vi "总磷氨氮测量流程.vi"(10 "量程模式":T1, 11 "参数":T2={"站号"=1, "量程切换"=enum."AUTO", "控制命令"=enum."启动测量", "模式设置"=enum."待机", "测量间隔"=0} {"站号" items=["总磷"=1, "总氮"=2]}) -> ()   [LabVIEW 2016]
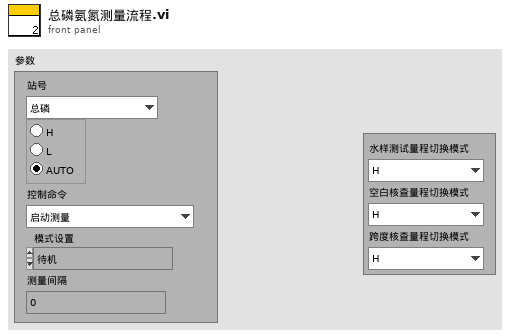
[diagram p1: front panel]
types:
  T1 = cluster{"水样测试量程切换模式":enum16{"H", "L", "AUTO"}, "空白核查量程切换模式":enum16{"H", "L", "AUTO"}, "跨度核查量程切换模式":enum16{"H", "L", "AUTO"}}
  T2 = cluster{"站号":u16, "量程切换":enum32{"H", "L", "AUTO"}, "控制命令":enum16{"启动测量", "标样核查", "零点核查", "跨度核查", "空白测试", "平行样测试", "加标回收", "空白校准", "标样校准", "初始化（清洗）", "停止测试", "仪器重启", "校时", "模式设置", "测量间隔设置"}, "模式设置":enum16{"待机", "连续模式", "周期模式", "定点模式", "受控模式", "手动模式"}, "测量间隔":u16}
  T3 = enum16{"初始化", "通电", "参数1启动", "等待参数1测试完成", "参数1测试完成", "参数1存储数据", "参数2启动", "等待参数2测试完成", "参数2测试完成", "参数2存储数据", "断电", "结束"}
  T4 = cluster{"时间标识":timestamp, "设备":string, "日志信息":string, "流程参数":string}
  T5 = cluster{"时间标识":timestamp, "监测值":sgl, "单位":u16, "数据标识":string, "因子编码":u32, "标样参考值":sgl, "F0":sgl, "F1":sgl, "F2":sgl, "F3":sgl, "温度":sgl, "湿度":sgl, "量程标识":string}
  T6 = enum16{"维护数据", "水样测试", "标样核查", "零点核查", "跨度核查", "空白测试", "平行样测试", "加标回收", "空白校准", "标样校准", "初始化（清洗）"}
  T7 = cluster{"系统时间":timestamp, "工作状态":enum16{"空闲", "水样测试", "标样核查", "零点核查", "跨度核查", "空白测试", "平行样测试", "加标回收", "空白校准", "标样校准", "初始化（清洗）"}, "测量模式":enum16{"待机", "连续模式", "周期模式", "定点模式", "受控模式", "手动模式"}, "告警代码":enum16{"无告警", "缺试剂告警", "缺水样告警", "缺蒸馏水告警", "缺标液告警", "仪表漏液告警", "标定异常告警", "超量程告警", "加热异常", "低试剂预警", "超上限告警", "超下限告警", "仪表内部其他异常", "滴定异常告警", "电极异常告警", "量程切换告警", "参数设置告警", "PH电极电位异常", "电导率电极异常", "浊度光度异常", "溶解氧电极异常", "溶解氧光强异常", "温度异常告警", "PH异常告警", "溶解氧异常告警", "电导率异常告警", "浊度异常告警", "叶绿素异常告警", "藻密度异常告警", "蓝绿藻异常告警", "ORP异常告警", "氨氮异常告警", "清洁刷异常告警", "SD卡异常告警", "蓝牙异常告警", "Wifi异常告警", "流程异常告警"}, "故障代码":enum16{"无故障", "电机故障", "温度故障", "通讯故障", "滴定故障"}, "日志代码":u16, "软件版本":u16, "F0":sgl, "F1":sgl, "F2":sgl, "F3":sgl, "T":sgl, "H":sgl, "id":u16, "flowid":u16, "量程":u16, "总磷控温温度1":sgl, "营养盐控温温度2":sgl, "ADC":sgl}
  T8 = enum16{"启动测量", "标样核查", "零点核查", "跨度核查", "空白测试", "平行样测试", "加标回收", "空白校准", "标样校准", "初始化（清洗）", "停止测试", "仪器重启", "校时", "模式设置", "测量间隔设置"}
  T9 = enum16{"空闲", "水样测试", "标样核查", "零点核查", "跨度核查", "空白测试", "平行样测试", "加标回收", "空白校准", "标样校准", "初始化（清洗）"}
  T10 = cluster{"因子编码":u32, "单位":u16, "标样参考值":sgl, "水样数据时间":timestamp, "水样实测值":sgl, "水样数据标识":string, "标样数据时间":timestamp, "标样实测值":sgl, "标样数据标识":string, "空白数据时间":timestamp, "空白实测值":sgl, "空白数据标识":string, "零点核查数据时间":timestamp, "零点核查实测值":sgl, "零点核查数据标识":string, "跨度核查数据时间":timestamp, "跨度核查实测值":sgl, "跨度核查数据标识":string, "加标回收数据时间":timestamp, "加标回收实测值":sgl, "加标回收数据标识":string, "平行样数据时间":timestamp, "平行样实测值":sgl, "平行样数据标识":string}
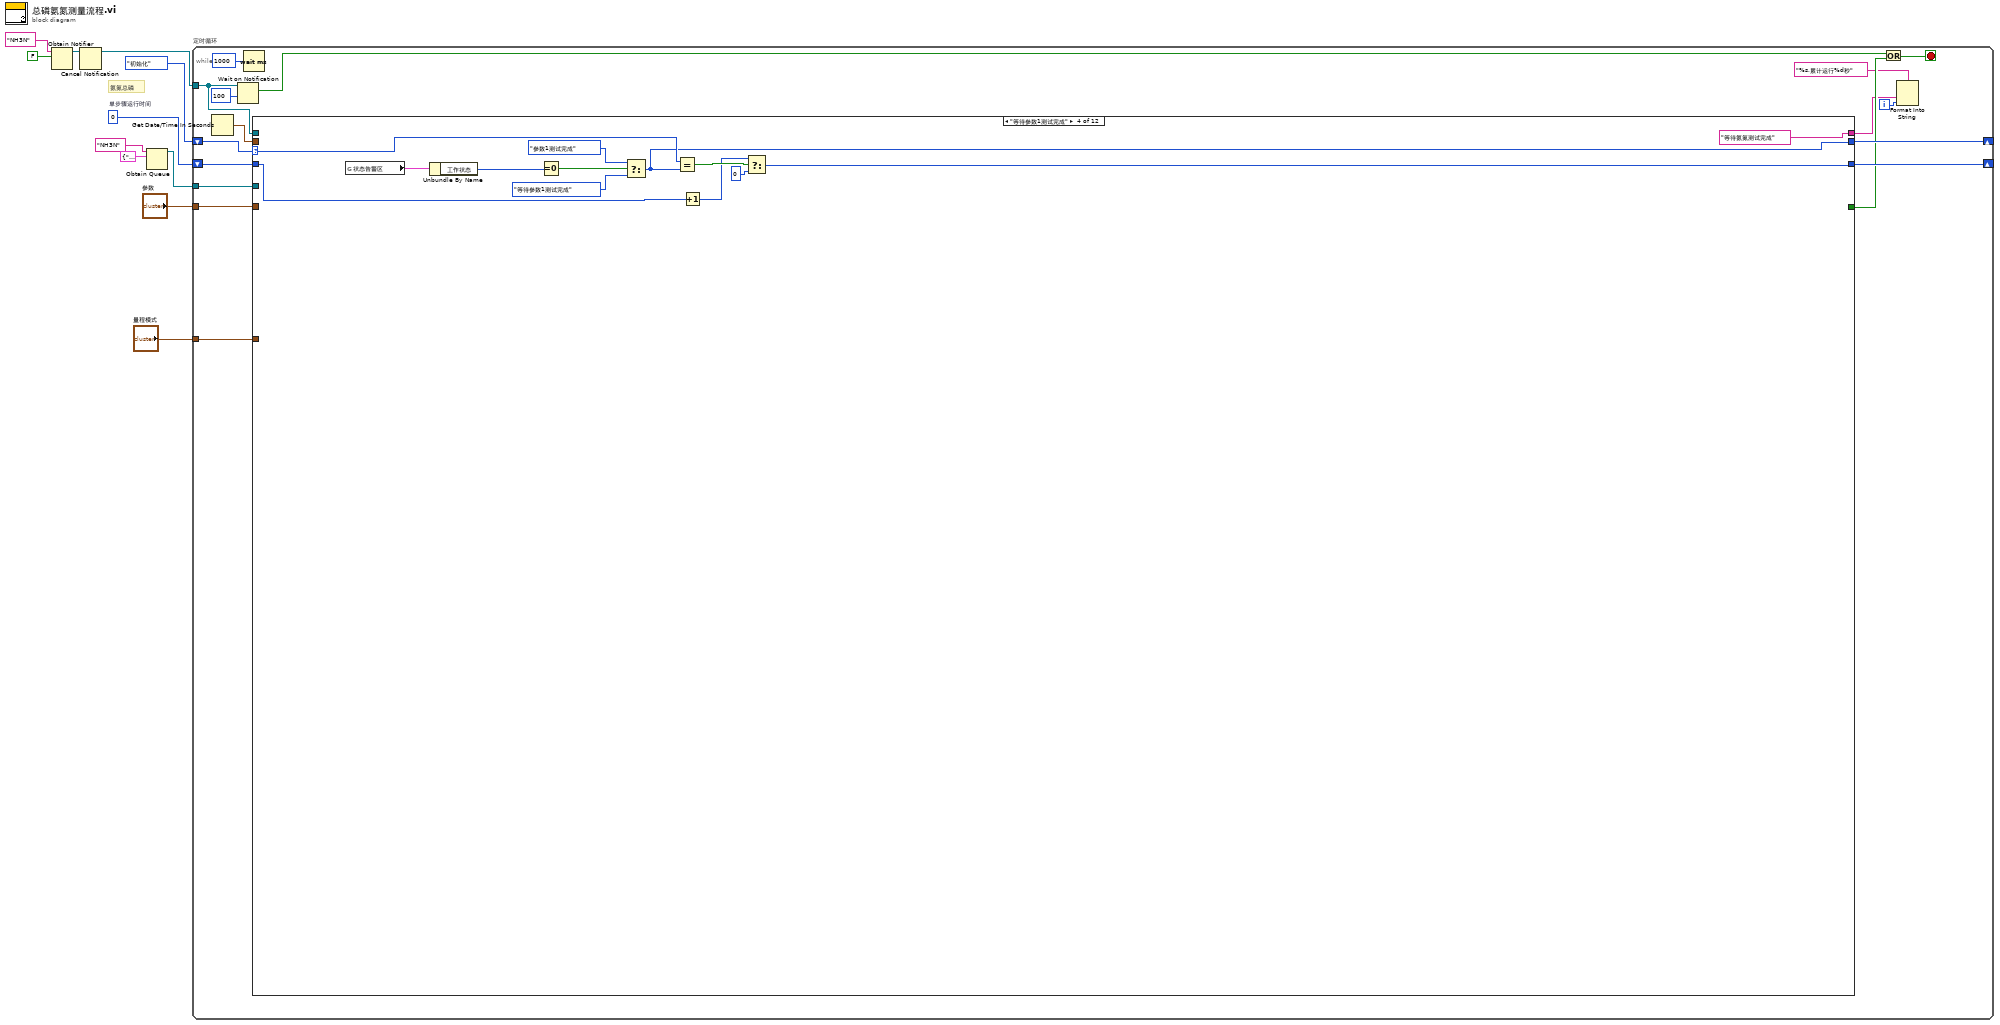
[diagram p0: block diagram]
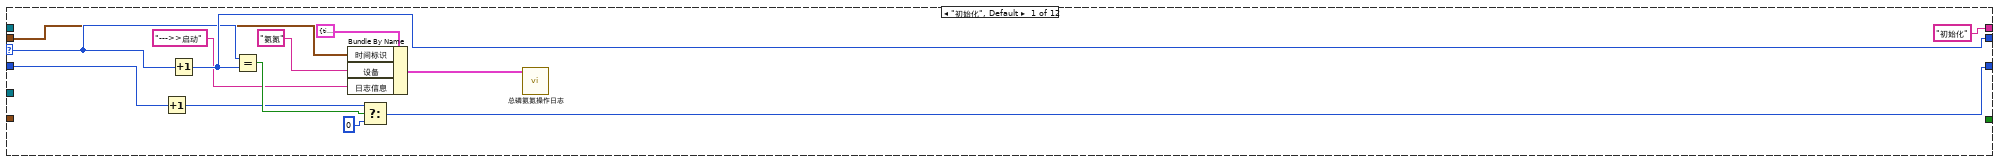
[diagram p2: hidden frame]
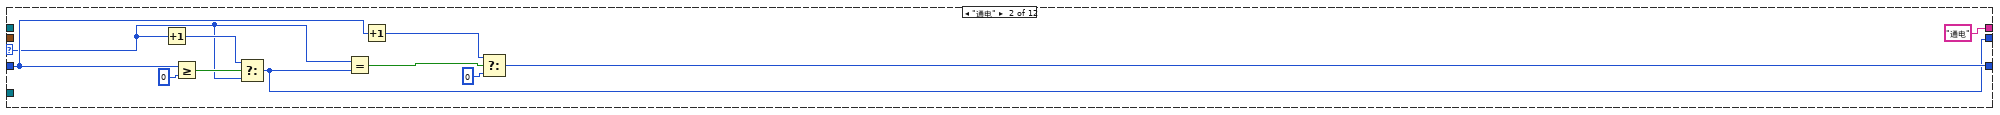
[diagram p3: hidden frame]
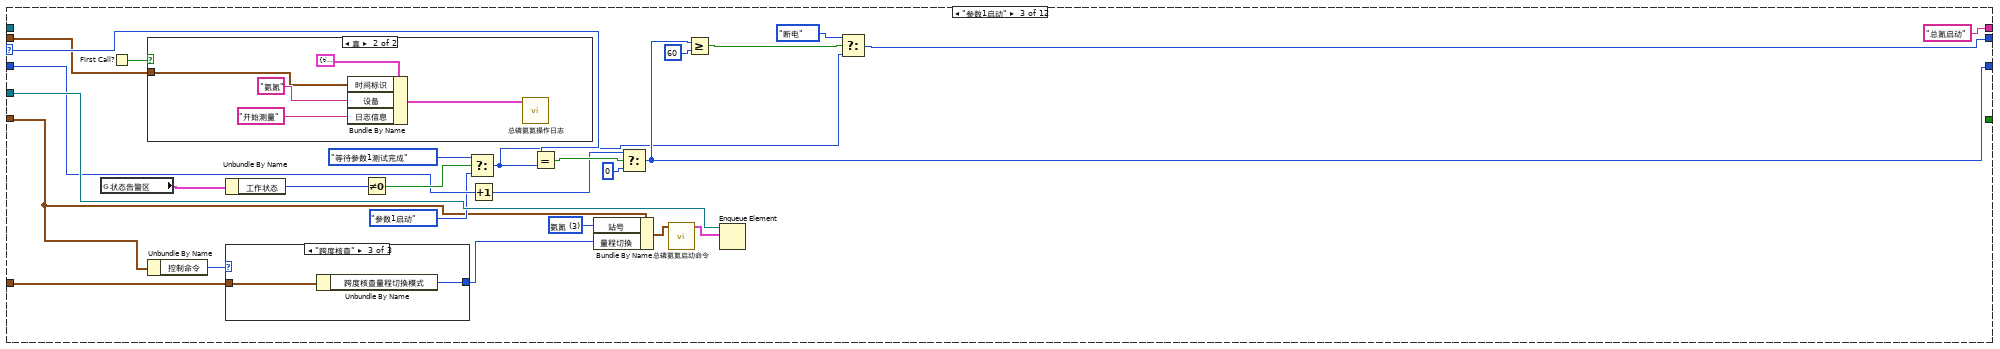
[diagram p4: hidden frame]
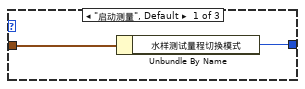
[diagram p5: hidden frame]
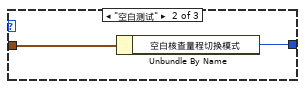
[diagram p6: hidden frame]
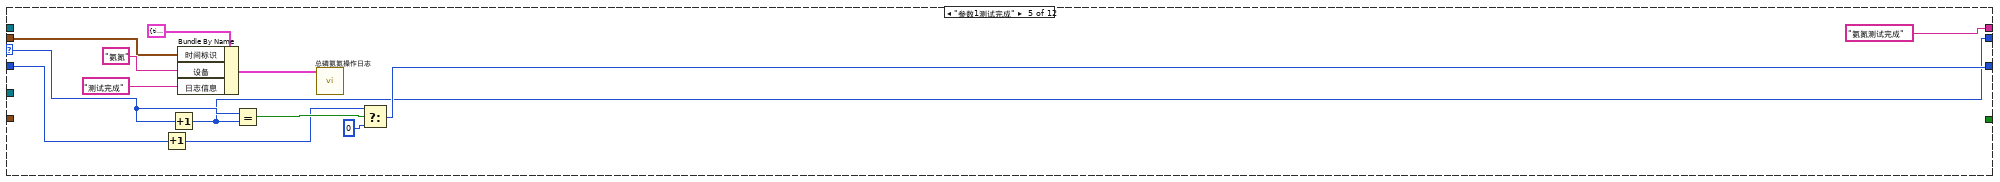
[diagram p8: hidden frame]
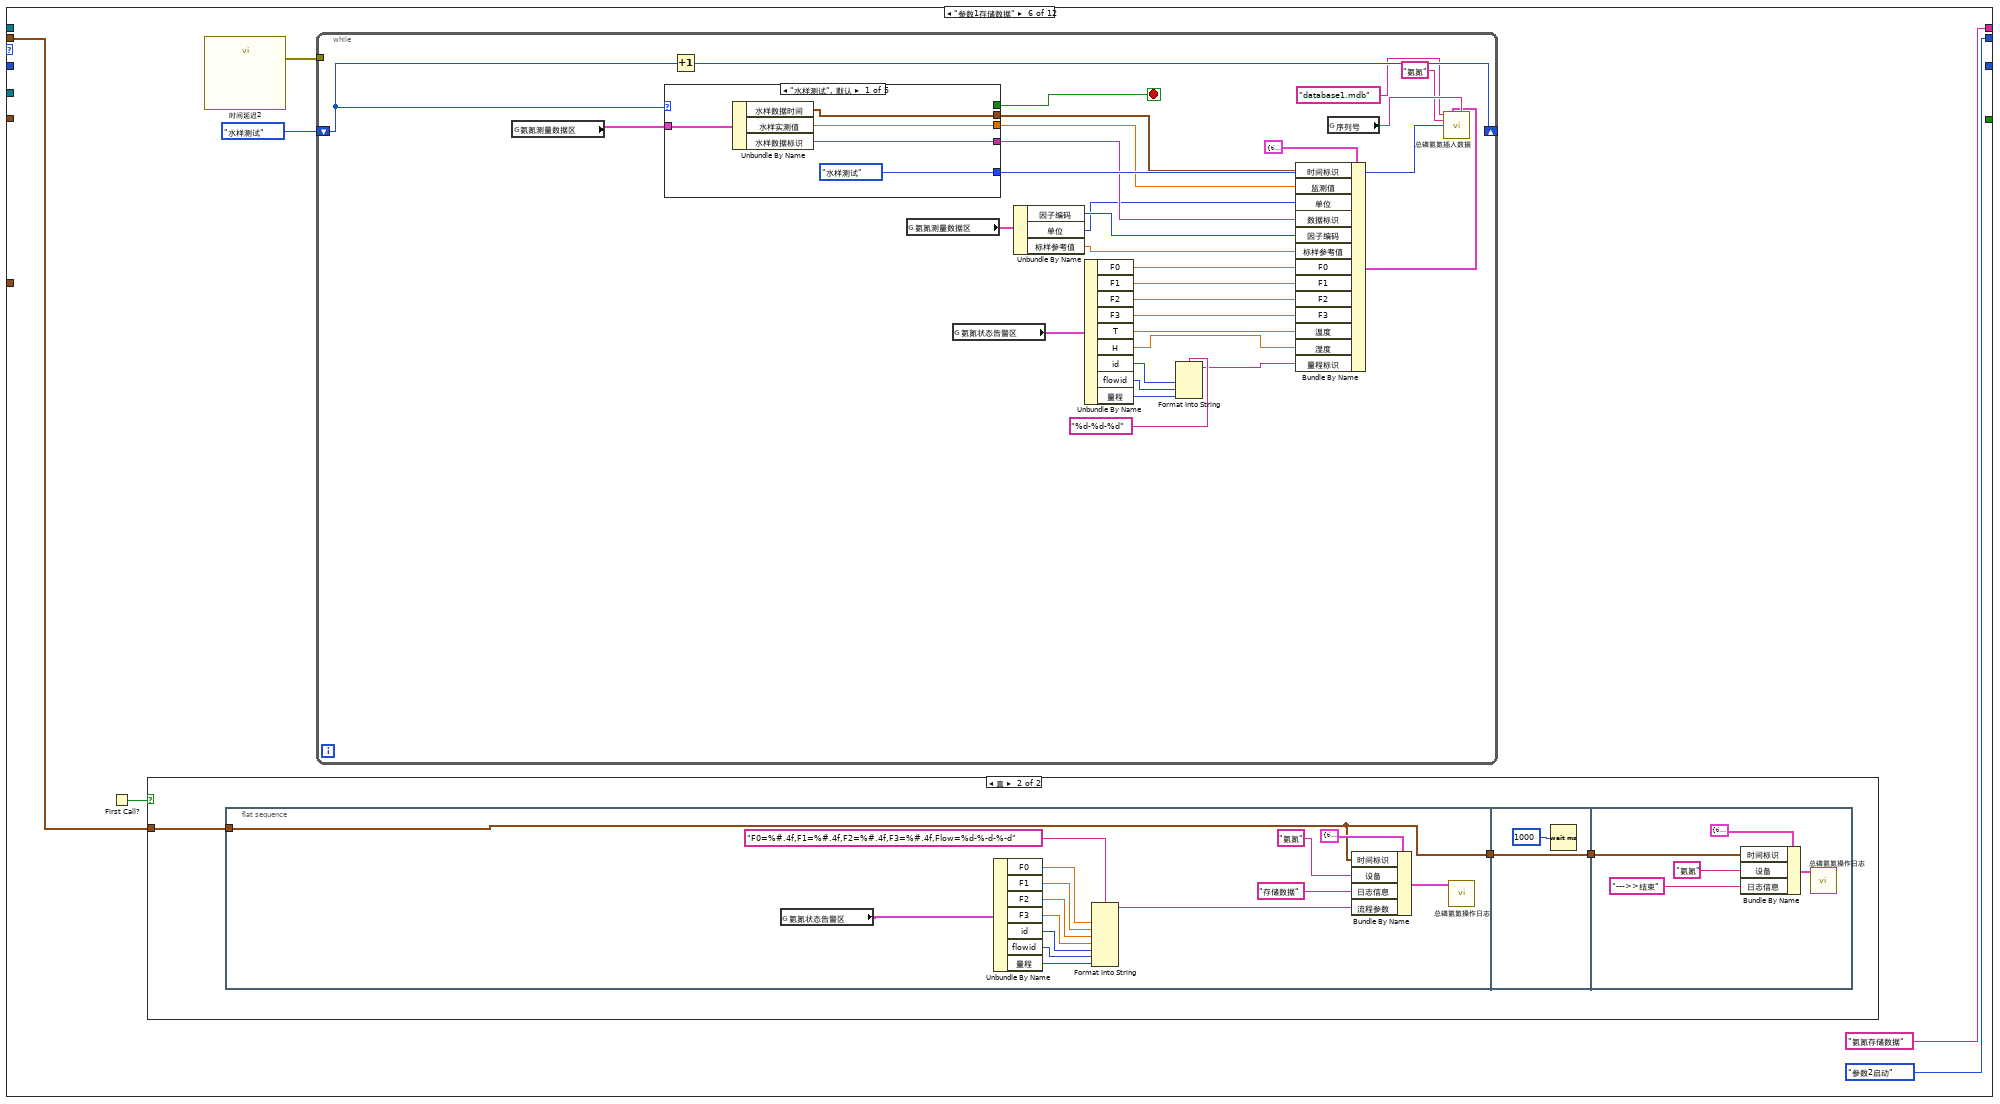
[diagram p9: hidden frame]
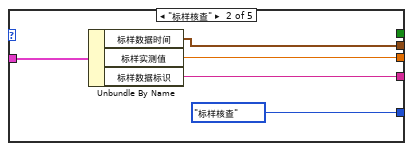
[diagram p10: hidden frame]
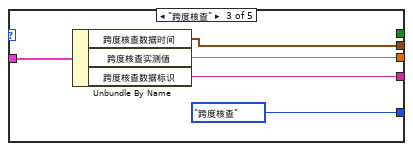
[diagram p11: hidden frame]
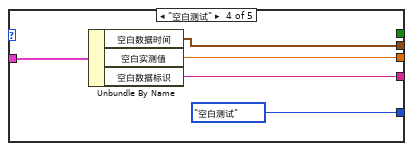
[diagram p12: hidden frame]
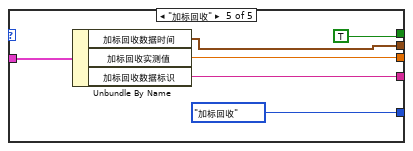
[diagram p13: hidden frame]
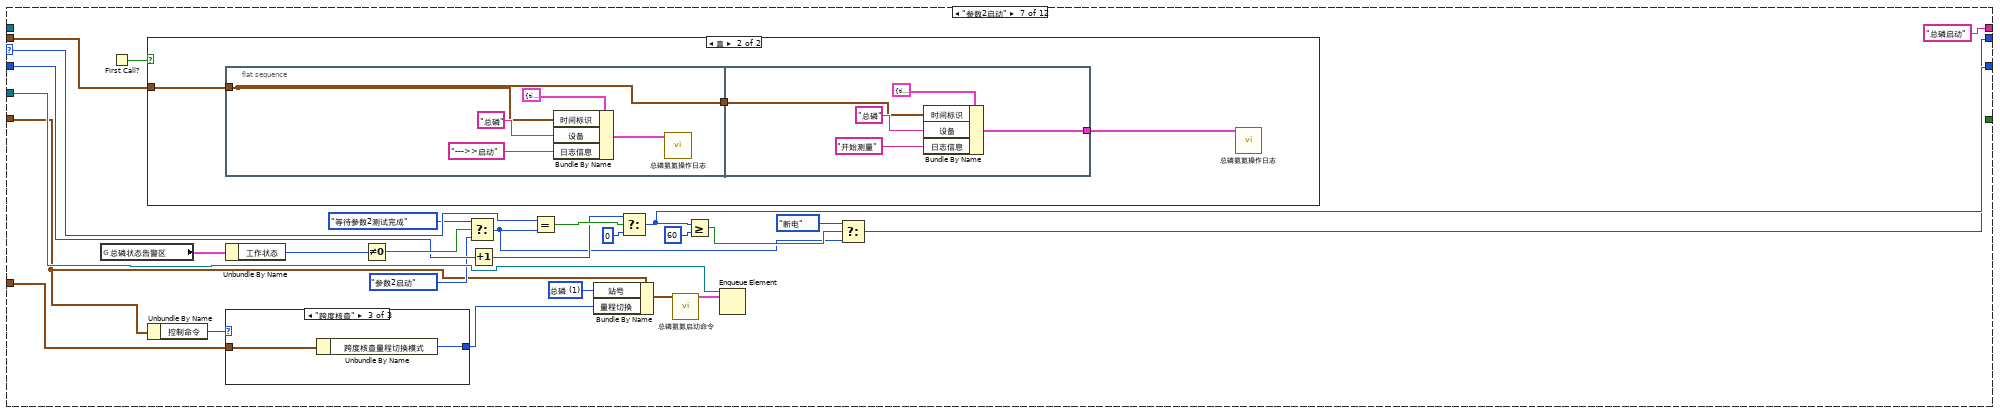
[diagram p15: hidden frame]
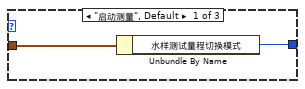
[diagram p16: hidden frame]
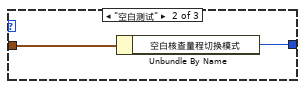
[diagram p17: hidden frame]
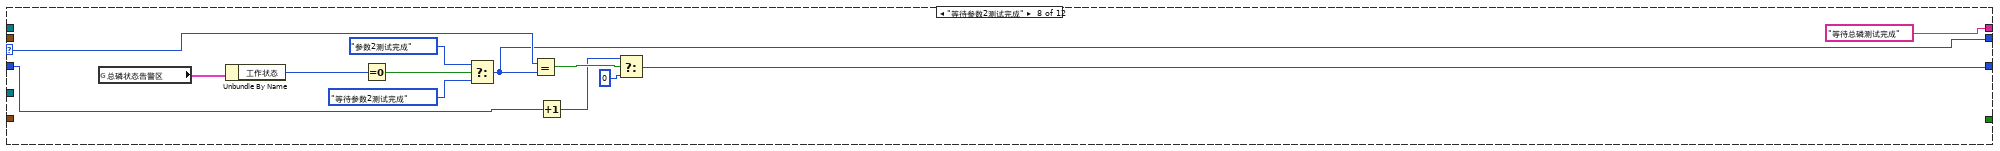
[diagram p19: hidden frame]
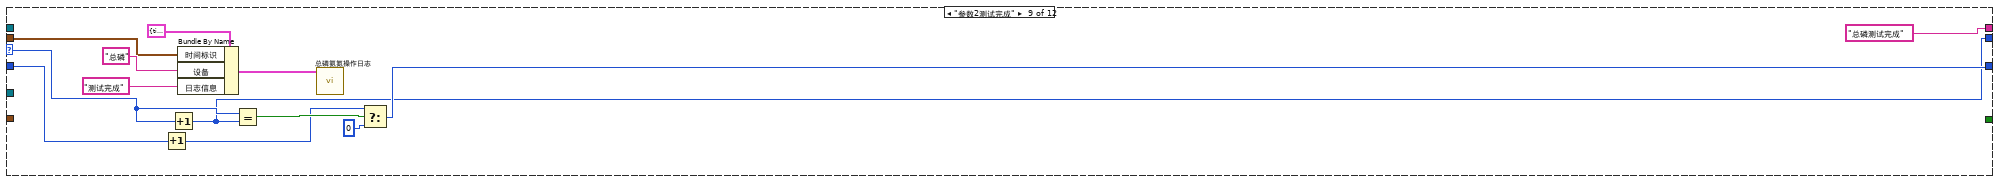
[diagram p20: hidden frame]
diagram:
  w8 = 0  # 单步骤运行时间
  # "氨氮总磷"
  n1 = Obtain Notifier(name (unnamed)="NH3N" ("名称（未命名）"), notification data type=FALSE) -> (notifier out=w6:refnum<notifier>)  [unwired: 2 in, 2 out]
  n2 = Cancel Notification(0:w6) -> (8:w5:refnum<notifier>)  [unwired: 1 in, 2 out]
  n3 = Obtain Queue(name (unnamed)="NH3N" ("名称（未命名）"), element data type=cluster{"命令":string, "data":variant} {"命令"="", "data"=variant}) -> (queue out=w9:refnum<queue>)  [unwired: 3 in, 2 out]
  n4 = while "定时循环" {
    shift-right: [w27] -> _
    shift-left: T3."初始化" ("枚举") -> [w28]
    tunnel: w9 -> [w26]
    shift-right: [w24] -> _
    shift-left: w8 -> [w25]
    tunnel: w5 -> [w23]
    tunnel: "参数" -> [w18]
    tunnel: "量程模式" -> [w12]
    i -> [w14]
    stop <- w19 stop-if-true
    n5 = Get Date/Time In Seconds() -> (seconds since 1Jan1904=w16:timestamp)
    n6 = Wait on Notification(notifier=w23, timeout in ms (-1)=100 ("超时毫秒(-1)")) -> (notification=w20:bool)  [unwired: 2 in, 3 out]
    n7 = Wait (ms)(milliseconds to wait=u32 1000 ("等待时间（毫秒）")) -> ()  [unwired: 1 out]
    n8 = case shown="\"等待参数1测试完成\"" w28 {
      selector: w28 -> [w39 w46 w74 w98 w113 _ w221 w255 w270 _ w357 _]
      tunnel: [_ _ _ _ _ _ _ _ _ _ _ TRUE] -> w21
      tunnel: [w40 w45 w56 w97 w112 T3."参数2启动" ("枚举") w206 w253 w268 T3."断电" ("枚举") w356 T3."结束" ("枚举")] -> w27
      tunnel: w26 -> [_ _ w79 _ _ _ w228 _ _ _ _ w369]
      tunnel: w25 -> [w41 w47 w75 w100 w114 _ w222 w256 w271 _ w359 _]
      tunnel: [w37 w48 w61 w99 w115 _ w207 w254 w269 0 ("t") w358 0 ("t")] -> w24
      tunnel: w23 -> [_ _ _ _ _ _ _ _ _ _ _ w368]
      tunnel: w18 -> [_ _ w65 _ _ _ w215 _ _ _ _ _]
      tunnel: w16 -> [w30 _ w70 _ w105 w122 w220 _ w263 w280 _ w362]
      tunnel: ["初始化" ("输入 1") "通电" ("输入 1") "总氮启动" ("输入 1") "等待氨氮测试完成" ("输入 1") "氨氮测试完成" ("输入 1") "氨氮存储数据" ("输入 1") "总磷启动" ("输入 1") "等待总磷测试完成" ("输入 1") "总磷测试完成" ("输入 1") "总磷存储数据" ("输入 1") "断电" ("输入 1") "结束" ("输入 1")] -> w13
      tunnel: w12 -> [_ _ w63 _ _ _ w213 _ _ _ _ _]
      frame "初始化", Default {
        n9 = Increment(x=w41) -> (x+1=w35:i32)
        n10 = Increment(x=w39) -> (x+1=w40:T3)
        n11 = Equal?(x=w39, y=w40) -> (x = y?=w38:bool)
        n12 = Bundle By Name(cluster=T4 {"时间标识"=timestamp(0 s since 1904-01-01), "设备"="", "日志信息"="", "流程参数"=""} ("data in"), "时间标识"=w30, "设备"="氨氮", "日志信息"="--->>启动") -> (w34:T4)
        n13 = Select(t=w35, s=w38, f=0 ("t")) -> (s? t:f=w37:i32)
        n14 = call "总磷氨氮操作日志.vi"("data in"=w34) -> ()  [unwired: 11 in]
      }
      frame "通电" {
        n15 = Increment(x=w46) -> (x+1=w50:T3)
        n16 = Greater Or Equal?(x=w47, y=0) -> (x >= y?=w51:bool)
        n17 = Select(t=w50, s=w51, f=w46) -> (s? t:f=w45:T3)
        n18 = Equal?(x=w46, y=w45) -> (x = y?=w49:bool)
        n19 = Increment(x=w47) -> (x+1=w44:i32)
        n20 = Select(t=w44, s=w49, f=0 ("t")) -> (s? t:f=w48:i32)
      }
      frame "参数1启动" {
        w71 = u16 3 items=["总磷"=1, "总氮"=2, "氨氮"=3] ("站号")
        n21 = global read "VAR总磷氨氮全局变量.vi" "状态告警区"() -> (w53:T7)
        n22 = First Call?() -> (First Call?: T/F=w69:bool)
        n23 = case shown="真" w69 {
          tunnel: w70 -> [_ w86]
          frame False {
          }
          frame True {
            n24 = Bundle By Name(cluster=T4 {"时间标识"=timestamp(0 s since 1904-01-01), "设备"="", "日志信息"="", "流程参数"=""} ("data in"), "时间标识"=w86, "设备"="氨氮", "日志信息"="开始测量") -> (w90:T4)
            n25 = call "总磷氨氮操作日志.vi"("data in"=w90) -> ()  [unwired: 11 in]
          }
        }
        n26 = Unbundle By Name(w65) -> ("控制命令"=w64:T8)
        n27 = Unbundle By Name(w53) -> ("工作状态"=w78:T9)
        n28 = case shown="\"跨度核查\"" w64 {
          tunnel: w63 -> [w81 w83 w85]
          tunnel: [w80 w82 w84] -> w62
          frame "启动测量", Default {
            n29 = Unbundle By Name(w81) -> ("水样测试量程切换模式"=w80:enum16{"H", "L", "AUTO"})
          }
          frame "空白测试" {
            n30 = Unbundle By Name(w83) -> ("空白核查量程切换模式"=w82:enum16{"H", "L", "AUTO"})
          }
          frame "跨度核查" {
            n31 = Unbundle By Name(w85) -> ("跨度核查量程切换模式"=w84:enum16{"H", "L", "AUTO"})
          }
        }
        n32 = Not Equal To 0?(x=w78) -> (x != 0?=w77:bool)
        n33 = Select(t=T3."等待参数1测试完成" ("枚举"), s=w77, f=T3."参数1启动" ("枚举")) -> (s? t:f=w58:T3)
        n34 = Increment(x=w75) -> (x+1=w72:i32)
        n35 = Equal?(x=w74, y=w58) -> (x = y?=w76:bool)
        n36 = Bundle By Name(cluster=w65, "站号"=w71, "量程切换"=w62) -> (w55:T2)
        n37 = Select(t=w72, s=w76, f=0 ("t")) -> (s? t:f=w61:i32)
        n38 = call "总磷氨氮启动命令.vi"("参数"=w55) -> ("启动命令"=w54:cluster{"命令":string, "data":variant})  [unwired: 10 in]
        n39 = Greater Or Equal?(x=w61, y=60) -> (x >= y?=w59:bool)
        n40 = Enqueue Element(queue=w79, element=w54) -> ()  [unwired: 2 in, 3 out]
        n41 = Select(t=T3."断电" ("枚举"), s=w59, f=w58) -> (s? t:f=w56:T3)
      }
      frame "等待参数1测试完成" {
        n42 = global read "VAR总磷氨氮全局变量.vi" "状态告警区"() -> (w91:T7)
        n43 = Unbundle By Name(w91) -> ("工作状态"=w103:T9)
        n44 = Equal To 0?(x=w103) -> (x = 0?=w102:bool)
        n45 = Select(t=T3."参数1测试完成" ("枚举"), s=w102, f=T3."等待参数1测试完成" ("枚举")) -> (s? t:f=w97:T3)
        n46 = Equal?(x=w98, y=w97) -> (x = y?=w101:bool)
        n47 = Increment(x=w100) -> (x+1=w95:i32)
        n48 = Select(t=w95, s=w101, f=0 ("t")) -> (s? t:f=w99:i32)
      }
      frame "参数1测试完成" {
        n49 = Increment(x=w114) -> (x+1=w110:i32)
        n50 = Increment(x=w113) -> (x+1=w112:T3)
        n51 = Bundle By Name(cluster=T4 {"时间标识"=timestamp(0 s since 1904-01-01), "设备"="", "日志信息"="", "流程参数"=""} ("data in"), "时间标识"=w105, "设备"="氨氮", "日志信息"="测试完成") -> (w109:T4)
        n52 = Equal?(x=w113, y=w112) -> (x = y?=w116:bool)
        n53 = call "总磷氨氮操作日志.vi"("data in"=w109) -> ()  [unwired: 11 in]
        n54 = Select(t=w110, s=w116, f=0 ("t")) -> (s? t:f=w115:i32)
      }
      frame "参数1存储数据" {
        n55 = First Call?() -> (First Call?: T/F=w120:bool)
        n56 = case shown="真" w120 {
          tunnel: w122 -> [_ w180]
          frame False {
          }
          frame True {
            n57 = flat-sequence {
              tunnel: w180 -> [w191]
              tunnel: [w191] -> w179
              tunnel: w179 -> [w197]
              tunnel: [w197] -> w178
              tunnel: w178 -> [w198]
              frame #0 {
                n58 = global read "VAR总磷氨氮全局变量.vi" "氨氮状态告警区"() -> (w181:T7)
                n59 = Unbundle By Name(w181) -> ("F0"=w183:sgl, "F1"=w184:sgl, "F2"=w185:sgl, "F3"=w186:sgl, "id"=w187:u16, "flowid"=w188:u16, "量程"=w189:u16)
                n60 = Format Into String(format string="F0=%#.4f,F1=%#.4f,F2=%#.4f,F3=%#.4f,Flow=%d-%-d-%-d" ("格式字符串"), w183, w184, w185, w186, w187, w188, w189) -> (resulting string=w182:string)  [unwired: 2 in, 1 out]
                n61 = Bundle By Name(cluster=T4 {"时间标识"=timestamp(0 s since 1904-01-01), "设备"="", "日志信息"="", "流程参数"=""} ("data in"), "时间标识"=w191, "设备"="氨氮", "日志信息"="存储数据", "流程参数"=w182) -> (w195:T4)
                n62 = call "总磷氨氮操作日志.vi"("data in"=w195) -> ()  [unwired: 11 in]
              }
              frame #1 {
                n63 = Wait (ms)(milliseconds to wait=u32 1000 ("等待时间（毫秒）")) -> ()  [unwired: 1 out]
              }
              frame #2 {
                n64 = Bundle By Name(cluster=T4 {"时间标识"=timestamp(0 s since 1904-01-01), "设备"="", "日志信息"="", "流程参数"=""} ("data in"), "时间标识"=w198, "设备"="氨氮", "日志信息"="--->>结束") -> (w199:T4)
                n65 = call "总磷氨氮操作日志.vi"("data in"=w199) -> ()  [unwired: 11 in]
              }
            }
          }
        }
        n66 = call "时间延迟2"() -> ("error out"=w117:errorcluster)  [unwired: 11 in]
        n67 = while {
          shift-right: [w149] -> _
          shift-left: enum16{"水样测试", "标样核查", "跨度核查", "空白测试", "加标回收"}."水样测试" ("测量模式") -> [w150]
          tunnel: w117 -> [_]
          stop <- w151 stop-if-true
          n68 = global read "VAR总磷氨氮全局变量.vi" "氨氮测量数据区"() -> (w148:T10)
          n69 = case shown="\"水样测试\", 默认" w150 {
            tunnel: w148 -> [w152 w157 w162 w167 w172]
            tunnel: [w156 w161 w166 w171 w177] -> w129
            tunnel: [w155 w160 w165 w170 w176] -> w128
            tunnel: [w154 w159 w164 w169 w175] -> w127
            tunnel: [T6."水样测试" ("测量模式") T6."标样核查" ("测量模式") T6."跨度核查" ("测量模式") T6."空白测试" ("测量模式") T6."加标回收" ("测量模式")] -> w144
            tunnel: [_ _ _ _ TRUE] -> w151
            frame "水样测试", Default {
              n70 = Unbundle By Name(w152) -> ("水样数据时间"=w156:timestamp, "水样实测值"=w155:sgl, "水样数据标识"=w154:string)
            }
            frame "标样核查" {
              n71 = Unbundle By Name(w157) -> ("标样数据时间"=w161:timestamp, "标样实测值"=w160:sgl, "标样数据标识"=w159:string)
            }
            frame "跨度核查" {
              n72 = Unbundle By Name(w162) -> ("跨度核查数据时间"=w166:timestamp, "跨度核查实测值"=w165:sgl, "跨度核查数据标识"=w164:string)
            }
            frame "空白测试" {
              n73 = Unbundle By Name(w167) -> ("空白数据时间"=w171:timestamp, "空白实测值"=w170:sgl, "空白数据标识"=w169:string)
            }
            frame "加标回收" {
              n74 = Unbundle By Name(w172) -> ("加标回收数据时间"=w177:timestamp, "加标回收实测值"=w176:sgl, "加标回收数据标识"=w175:string)
            }
          }
          n75 = Increment(x=w150) -> (x+1=w149:enum16{"水样测试", "标样核查", "跨度核查", "空白测试", "加标回收"})
          n76 = global read "VAR总磷氨氮全局变量.vi" "氨氮测量数据区"() -> (w126:T10)
          n77 = global read "VAR总磷氨氮全局变量.vi" "氨氮状态告警区"() -> (w143:T7)
          n78 = Unbundle By Name(w126) -> ("因子编码"=w125:u32, "单位"=w124:u16, "标样参考值"=w123:sgl)
          n79 = Unbundle By Name(w143) -> ("F0"=w142:sgl, "F1"=w141:sgl, "F2"=w140:sgl, "F3"=w139:sgl, "T"=w138:sgl, "H"=w137:sgl, "id"=w135:u16, "flowid"=w134:u16, "量程"=w133:u16)
          n80 = Format Into String(format string="%d-%d-%d" ("格式字符串"), w135, w134, w133) -> (resulting string=w131:string)  [unwired: 2 in, 1 out]
          n81 = Bundle By Name(cluster=T5 {"时间标识"=timestamp(0 s since 1904-01-01), "监测值"=0.0, "单位"=0, "数据标识"="", "因子编码"=0, "标样参考值"=0.0, "F0"=0.0, "F1"=0.0, "F2"=0.0, "F3"=0.0, "温度"=0.0, "湿度"=0.0, "量程标识"=""} ("data"), "时间标识"=w129, "监测值"=w128, "单位"=w124, "数据标识"=w127, "因子编码"=w125, "标样参考值"=w123, "F0"=w142, "F1"=w141, "F2"=w140, "F3"=w139, "温度"=w138, "湿度"=w137, "量程标识"=w131) -> (w130:T5)
          n82 = global read "VAR总磷氨氮全局变量.vi" "序列号"() -> (w147:string)
          n83 = call "总磷氨氮插入数据.vi"("database"="database1.mdb", "data"=w130, "SN"=w147, "table"="氨氮", "测量模式"=w144) -> ()  [unwired: 10 in, 1 out]
        }
      }
      frame "参数2启动" {
        w229 = u16 1 items=["总氮"=2, "总磷"=1] ("站号")
        n84 = global read "VAR总磷氨氮全局变量.vi" "总磷状态告警区"() -> (w205:T7)
        n85 = First Call?() -> (First Call?: T/F=w219:bool)
        n86 = case shown="真" w219 {
          tunnel: w220 -> [_ w236]
          frame False {
          }
          frame True {
            n87 = flat-sequence {
              tunnel: w236 -> [w239]
              tunnel: [w239] -> w237
              tunnel: [w248] -> w238
              tunnel: w237 -> [w244]
              frame #0 {
                n88 = Bundle By Name(cluster=T4 {"时间标识"=timestamp(0 s since 1904-01-01), "设备"="", "日志信息"="", "流程参数"=""} ("data in"), "时间标识"=w239, "设备"="总磷", "日志信息"="--->>启动") -> (w243:T4)
                n89 = call "总磷氨氮操作日志.vi"("data in"=w243) -> ()  [unwired: 11 in]
              }
              frame #1 {
                n90 = Bundle By Name(cluster=T4 {"时间标识"=timestamp(0 s since 1904-01-01), "设备"="", "日志信息"="", "流程参数"=""} ("data in"), "时间标识"=w244, "设备"="总磷", "日志信息"="开始测量") -> (w248:T4)
              }
            }
            n91 = call "总磷氨氮操作日志.vi"("data in"=w238) -> ()  [unwired: 11 in]
          }
        }
        n92 = Unbundle By Name(w215) -> ("控制命令"=w214:T8)
        n93 = Unbundle By Name(w205) -> ("工作状态"=w227:T9)
        n94 = case shown="\"跨度核查\"" w214 {
          tunnel: w213 -> [w231 w233 w235]
          tunnel: [w230 w232 w234] -> w212
          frame "启动测量", Default {
            n95 = Unbundle By Name(w231) -> ("水样测试量程切换模式"=w230:enum16{"H", "L", "AUTO"})
          }
          frame "空白测试" {
            n96 = Unbundle By Name(w233) -> ("空白核查量程切换模式"=w232:enum16{"H", "L", "AUTO"})
          }
          frame "跨度核查" {
            n97 = Unbundle By Name(w235) -> ("跨度核查量程切换模式"=w234:enum16{"H", "L", "AUTO"})
          }
        }
        n98 = Not Equal To 0?(x=w227) -> (x != 0?=w226:bool)
        n99 = Select(t=T3."等待参数2测试完成" ("枚举"), s=w226, f=T3."参数2启动" ("枚举")) -> (s? t:f=w208:T3)
        n100 = Increment(x=w222) -> (x+1=w223:i32)
        n101 = Equal?(x=w221, y=w208) -> (x = y?=w225:bool)
        n102 = Bundle By Name(cluster=w215, "站号"=w229, "量程切换"=w212) -> (w204:T2)
        n103 = Select(t=w223, s=w225, f=0 ("t")) -> (s? t:f=w207:i32)
        n104 = call "总磷氨氮启动命令.vi"("参数"=w204) -> ("启动命令"=w203:cluster{"命令":string, "data":variant})  [unwired: 10 in]
        n105 = Greater Or Equal?(x=w207, y=60) -> (x >= y?=w210:bool)
        n106 = Enqueue Element(queue=w228, element=w203) -> ()  [unwired: 2 in, 3 out]
        n107 = Select(t=T3."断电" ("枚举"), s=w210, f=w208) -> (s? t:f=w206:T3)
      }
      frame "等待参数2测试完成" {
        n108 = global read "VAR总磷氨氮全局变量.vi" "总磷状态告警区"() -> (w249:T7)
        n109 = Unbundle By Name(w249) -> ("工作状态"=w261:T9)
        n110 = Equal To 0?(x=w261) -> (x = 0?=w260:bool)
        n111 = Select(t=T3."参数2测试完成" ("枚举"), s=w260, f=T3."等待参数2测试完成" ("枚举")) -> (s? t:f=w253:T3)
        n112 = Equal?(x=w255, y=w253) -> (x = y?=w259:bool)
        n113 = Increment(x=w256) -> (x+1=w257:i32)
        n114 = Select(t=w257, s=w259, f=0 ("t")) -> (s? t:f=w254:i32)
      }
      frame "参数2测试完成" {
        n115 = Increment(x=w271) -> (x+1=w272:i32)
        n116 = Increment(x=w270) -> (x+1=w268:T3)
        n117 = Bundle By Name(cluster=T4 {"时间标识"=timestamp(0 s since 1904-01-01), "设备"="", "日志信息"="", "流程参数"=""} ("data in"), "时间标识"=w263, "设备"="总磷", "日志信息"="测试完成") -> (w267:T4)
        n118 = Equal?(x=w270, y=w268) -> (x = y?=w274:bool)
        n119 = call "总磷氨氮操作日志.vi"("data in"=w267) -> ()  [unwired: 11 in]
        n120 = Select(t=w272, s=w274, f=0 ("t")) -> (s? t:f=w269:i32)
      }
      frame "参数2存储数据" {
        n121 = First Call?() -> (First Call?: T/F=w277:bool)
        n122 = case shown="真" w277 {
          tunnel: w280 -> [_ w347]
          frame False {
          }
          frame True {
            n123 = global read "VAR总磷氨氮全局变量.vi" "总磷状态告警区"() -> (w337:T7)
            n124 = Unbundle By Name(w337) -> ("F0"=w339:sgl, "F1"=w340:sgl, "F2"=w341:sgl, "F3"=w342:sgl, "id"=w343:u16, "flowid"=w344:u16, "量程"=w345:u16)
            n125 = Format Into String(format string="F0=%#.4f,F1=%#.4f,F2=%#.4f,F3=%#.4f,Flow=%d-%-d-%-d" ("格式字符串"), w339, w340, w341, w342, w343, w344, w345) -> (resulting string=w338:string)  [unwired: 2 in, 1 out]
            n126 = Bundle By Name(cluster=T4 {"时间标识"=timestamp(0 s since 1904-01-01), "设备"="", "日志信息"="", "流程参数"=""} ("data in"), "时间标识"=w347, "设备"="总磷", "日志信息"="存储数据", "流程参数"=w338) -> (w351:T4)
            n127 = call "总磷氨氮操作日志.vi"("data in"=w351) -> ()  [unwired: 11 in]
          }
        }
        n128 = call "时间延迟"() -> ("error out"=w275:errorcluster)  [unwired: 11 in]
        n129 = while {
          shift-right: [w308] -> _
          shift-left: enum16{"水样测试", "标样核查", "跨度核查", "空白测试", "加标回收"}."水样测试" ("测量模式") -> [w309]
          tunnel: w275 -> [_]
          stop <- w310 stop-if-true
          n130 = global read "VAR总磷氨氮全局变量.vi" "总磷测量数据区"() -> (w307:T10)
          n131 = case shown="\"空白测试\"" w309 {
            tunnel: w307 -> [w315 w320 w325 w330 w336]
            tunnel: [w314 w319 w324 w329 w335] -> w300
            tunnel: [w313 w318 w323 w328 w334] -> w299
            tunnel: [w312 w317 w322 w327 w333] -> w298
            tunnel: [T6."水样测试" ("测量模式") T6."标样核查" ("测量模式") T6."跨度核查" ("测量模式") T6."空白测试" ("测量模式") T6."加标回收" ("测量模式")] -> w304
            tunnel: [_ _ _ _ TRUE] -> w310
            frame "水样测试", Default {
              n132 = Unbundle By Name(w315) -> ("水样数据时间"=w314:timestamp, "水样实测值"=w313:sgl, "水样数据标识"=w312:string)
            }
            frame "标样核查" {
              n133 = Unbundle By Name(w320) -> ("标样数据时间"=w319:timestamp, "标样实测值"=w318:sgl, "标样数据标识"=w317:string)
            }
            frame "跨度核查" {
              n134 = Unbundle By Name(w325) -> ("跨度核查数据时间"=w324:timestamp, "跨度核查实测值"=w323:sgl, "跨度核查数据标识"=w322:string)
            }
            frame "空白测试" {
              n135 = Unbundle By Name(w330) -> ("空白数据时间"=w329:timestamp, "空白实测值"=w328:sgl, "空白数据标识"=w327:string)
            }
            frame "加标回收" {
              n136 = Unbundle By Name(w336) -> ("加标回收数据时间"=w335:timestamp, "加标回收实测值"=w334:sgl, "加标回收数据标识"=w333:string)
            }
          }
          n137 = Increment(x=w309) -> (x+1=w308:enum16{"水样测试", "标样核查", "跨度核查", "空白测试", "加标回收"})
          n138 = global read "VAR总磷氨氮全局变量.vi" "总磷测量数据区"() -> (w285:T10)
          n139 = global read "VAR总磷氨氮全局变量.vi" "总磷状态告警区"() -> (w297:T7)
          n140 = Unbundle By Name(w285) -> ("因子编码"=w284:u32, "单位"=w283:u16, "标样参考值"=w282:sgl)
          n141 = Unbundle By Name(w297) -> ("F0"=w292:sgl, "F1"=w291:sgl, "F2"=w290:sgl, "F3"=w289:sgl, "T"=w288:sgl, "H"=w287:sgl, "id"=w295:u16, "flowid"=w294:u16, "量程"=w293:u16)
          n142 = Format Into String(format string="%d-%d-%d" ("格式字符串"), w295, w294, w293) -> (resulting string=w286:string)  [unwired: 2 in, 1 out]
          n143 = Bundle By Name(cluster=T5 {"时间标识"=timestamp(0 s since 1904-01-01), "监测值"=0.0, "单位"=0, "数据标识"="", "因子编码"=0, "标样参考值"=0.0, "F0"=0.0, "F1"=0.0, "F2"=0.0, "F3"=0.0, "温度"=0.0, "湿度"=0.0, "量程标识"=""} ("data"), "时间标识"=w300, "监测值"=w299, "单位"=w283, "数据标识"=w298, "因子编码"=w284, "标样参考值"=w282, "F0"=w292, "F1"=w291, "F2"=w290, "F3"=w289, "温度"=w288, "湿度"=w287, "量程标识"=w286) -> (w301:T5)
          n144 = global read "VAR总磷氨氮全局变量.vi" "序列号"() -> (w303:string)
          n145 = call "总磷氨氮插入数据.vi"("database"="database1.mdb", "data"=w301, "SN"=w303, "table"="总磷", "测量模式"=w304) -> ()  [unwired: 10 in, 1 out]
        }
      }
      frame "断电" {
        n146 = Increment(x=w359) -> (x+1=w352:i32)
        n147 = Increment(x=w357) -> (x+1=w356:T3)
        n148 = Equal?(x=w357, y=w356) -> (x = y?=w354:bool)
        n149 = Select(t=w352, s=w354, f=0 ("t")) -> (s? t:f=w358:i32)
      }
      frame "结束" {
        n150 = Release Queue(queue=w369) -> ()  [unwired: 2 in, 3 out]
        n151 = Cancel Notification(0:w368) -> (8:w367:refnum<notifier>)  [unwired: 1 in, 2 out]
        n152 = Release Notifier(notifier=w367) -> ()  [unwired: 2 in, 3 out]
        n153 = Bundle By Name(cluster=T4 {"时间标识"=timestamp(0 s since 1904-01-01), "设备"="", "日志信息"="", "流程参数"=""} ("data in"), "时间标识"=w362, "设备"="总磷", "日志信息"="--->>结束") -> (w366:T4)
        n154 = call "总磷氨氮操作日志.vi"("data in"=w366) -> ()  [unwired: 11 in]
      }
    }
    n155 = Or(x=w20, y=w21) -> (x .or. y?=w19:bool)
    n156 = Format Into String(format string="%s,累计运行%d秒" ("格式字符串"), w13, w14) -> ()  [unwired: 2 in, 2 out]
  }
